vi "メイン.vi"() -> (2 "測定周期/ms":dbl, 3 "値転記用配列":T2[](array[typedef]))   [LabVIEW 2021] (continued)
                          # "csv作成の為表へクラスタ(実測値)書き込み"
                          # "⑤"
                          # "③"
                          # "④"
                          n3514 = local read "メインON/OFF_\n設定 7"() -> (w6014:T1)
                          n3515 = Unbundle By Name(w6014) -> ("使用ON/OFF"=w6010:bool)
                          n3516 = control-ref of="前回値転記用配列"() -> (w6008:refnum<vi>)
                          n3517 = local read "メイン設定_設定 7"() -> (w6015:T2)
                          n3518 = call "メイン_測定値配列_CSV転記サブ.vi"("メイン設定_設定入力"=w6015, "ループ反復数値入力"=w6012, "実測設定項目"=w6013, "使用ON/OFF"=w6010, "前回値転記用配列"=w6008) -> ("ループ反復数値出力"=w6011:i32, "メイン設定_設定出力"=w6009:T2)  [unwired: 5 in]
                          n3519 = local write "メイン設定_設定 7"(w6009) -> ()
                          n3520 = Add(x=8, y=w6011) -> (x+y=w6004:i32)
                          n3521 = Add(x=w6011, y=9) -> (x+y=w6002:i32)
                          n3522 = local read "csv作成表"() -> (w5998:string[][])
                          n3523 = Unbundle By Name(w6009) -> ("実測値(MAX)"=w6005:string, "実測値(MIN)"=w6006:string)
                          n3524 = Replace Array Subset(array=w5998, new element #1=w6005, index (row) #1=w6003, index (col) #1=w6004, new element #2=w6006, index (row) #2=w6003, index (col) #2=w6002) -> (w6000:string[][])
                          n3525 = Select(t=w6000, s=w6010, f=w5998) -> (s? t:f=w6001:string[][])
                          n3526 = local write "csv作成表"(w6001) -> ()
                        }
                        frame 7 {
                          w6021 = 2
                          # "B"
                          # "A"
                          # "csv作成の為表へクラスタ(実測値)書き込み"
                          # "⑤"
                          # "③"
                          # "④"
                          n3527 = local read "メインON/OFF_\n設定 8"() -> (w6032:T1)
                          n3528 = Unbundle By Name(w6032) -> ("使用ON/OFF"=w6028:bool)
                          n3529 = control-ref of="前回値転記用配列"() -> (w6026:refnum<vi>)
                          n3530 = local read "メイン設定_設定 8"() -> (w6033:T2)
                          n3531 = call "メイン_測定値配列_CSV転記サブ.vi"("メイン設定_設定入力"=w6033, "ループ反復数値入力"=w6030, "実測設定項目"=w6031, "使用ON/OFF"=w6028, "前回値転記用配列"=w6026) -> ("ループ反復数値出力"=w6029:i32, "メイン設定_設定出力"=w6027:T2)  [unwired: 5 in]
                          n3532 = local write "メイン設定_設定 8"(w6027) -> ()
                          n3533 = Add(x=9, y=w6029) -> (x+y=w6022:i32)
                          n3534 = Add(x=w6029, y=10) -> (x+y=w6020:i32)
                          n3535 = local read "csv作成表"() -> (w6016:string[][])
                          n3536 = Unbundle By Name(w6027) -> ("実測値(MAX)"=w6023:string, "実測値(MIN)"=w6024:string)
                          n3537 = Replace Array Subset(array=w6016, new element #1=w6023, index (row) #1=w6021, index (col) #1=w6022, new element #2=w6024, index (row) #2=w6021, index (col) #2=w6020) -> (w6018:string[][])
                          n3538 = Select(t=w6018, s=w6028, f=w6016) -> (s? t:f=w6019:string[][])
                          n3539 = local write "csv作成表"(w6019) -> ()
                        }
                        frame 8 {
                          w6039 = 2
                          # "B"
                          # "A"
                          # "csv作成の為表へクラスタ(実測値)書き込み"
                          # "⑤"
                          # "③"
                          # "④"
                          n3540 = local read "メインON/OFF_\n設定 9"() -> (w6050:T1)
                          n3541 = Unbundle By Name(w6050) -> ("使用ON/OFF"=w6046:bool)
                          n3542 = control-ref of="前回値転記用配列"() -> (w6044:refnum<vi>)
                          n3543 = local read "メイン設定_設定 9"() -> (w6051:T2)
                          n3544 = call "メイン_測定値配列_CSV転記サブ.vi"("メイン設定_設定入力"=w6051, "ループ反復数値入力"=w6048, "実測設定項目"=w6049, "使用ON/OFF"=w6046, "前回値転記用配列"=w6044) -> ("ループ反復数値出力"=w6047:i32, "メイン設定_設定出力"=w6045:T2)  [unwired: 5 in]
                          n3545 = local write "メイン設定_設定 9"(w6045) -> ()
                          n3546 = Add(x=10, y=w6047) -> (x+y=w6040:i32)
                          n3547 = Add(x=w6047, y=11) -> (x+y=w6038:i32)
                          n3548 = local read "csv作成表"() -> (w6034:string[][])
                          n3549 = Unbundle By Name(w6045) -> ("実測値(MAX)"=w6041:string, "実測値(MIN)"=w6042:string)
                          n3550 = Replace Array Subset(array=w6034, new element #1=w6041, index (row) #1=w6039, index (col) #1=w6040, new element #2=w6042, index (row) #2=w6039, index (col) #2=w6038) -> (w6036:string[][])
                          n3551 = Select(t=w6036, s=w6046, f=w6034) -> (s? t:f=w6037:string[][])
                          n3552 = local write "csv作成表"(w6037) -> ()
                        }
                        frame 9 {
                          w6057 = 2
                          # "B"
                          # "A"
                          # "csv作成の為表へクラスタ(実測値)書き込み"
                          # "⑤"
                          # "③"
                          # "④"
                          n3553 = local read "メインON/OFF_\n設定 10"() -> (w6068:T1)
                          n3554 = Unbundle By Name(w6068) -> ("使用ON/OFF"=w6064:bool)
                          n3555 = control-ref of="前回値転記用配列"() -> (w6062:refnum<vi>)
                          n3556 = local read "メイン設定_設定 10"() -> (w6069:T2)
                          n3557 = call "メイン_測定値配列_CSV転記サブ.vi"("メイン設定_設定入力"=w6069, "ループ反復数値入力"=w6066, "実測設定項目"=w6067, "使用ON/OFF"=w6064, "前回値転記用配列"=w6062) -> ("ループ反復数値出力"=w6065:i32, "メイン設定_設定出力"=w6063:T2)  [unwired: 5 in]
                          n3558 = local write "メイン設定_設定 10"(w6063) -> ()
                          n3559 = Add(x=11, y=w6065) -> (x+y=w6058:i32)
                          n3560 = Add(x=w6065, y=12) -> (x+y=w6056:i32)
                          n3561 = local read "csv作成表"() -> (w6052:string[][])
                          n3562 = Unbundle By Name(w6063) -> ("実測値(MAX)"=w6059:string, "実測値(MIN)"=w6060:string)
                          n3563 = Replace Array Subset(array=w6052, new element #1=w6059, index (row) #1=w6057, index (col) #1=w6058, new element #2=w6060, index (row) #2=w6057, index (col) #2=w6056) -> (w6054:string[][])
                          n3564 = Select(t=w6054, s=w6064, f=w6052) -> (s? t:f=w6055:string[][])
                          n3565 = local write "csv作成表"(w6055) -> ()
                        }
                        frame 10 {
                          w6075 = 2
                          # "B"
                          # "A"
                          # "csv作成の為表へクラスタ(実測値)書き込み"
                          # "⑤"
                          # "③"
                          # "④"
                          n3566 = local read "メインON/OFF_\n設定 11"() -> (w6086:T1)
                          n3567 = Unbundle By Name(w6086) -> ("使用ON/OFF"=w6082:bool)
                          n3568 = control-ref of="前回値転記用配列"() -> (w6080:refnum<vi>)
                          n3569 = local read "メイン設定_設定 11"() -> (w6087:T2)
                          n3570 = call "メイン_測定値配列_CSV転記サブ.vi"("メイン設定_設定入力"=w6087, "ループ反復数値入力"=w6084, "実測設定項目"=w6085, "使用ON/OFF"=w6082, "前回値転記用配列"=w6080) -> ("ループ反復数値出力"=w6083:i32, "メイン設定_設定出力"=w6081:T2)  [unwired: 5 in]
                          n3571 = local write "メイン設定_設定 11"(w6081) -> ()
                          n3572 = Add(x=12, y=w6083) -> (x+y=w6076:i32)
                          n3573 = Add(x=w6083, y=13) -> (x+y=w6074:i32)
                          n3574 = local read "csv作成表"() -> (w6070:string[][])
                          n3575 = Unbundle By Name(w6081) -> ("実測値(MAX)"=w6077:string, "実測値(MIN)"=w6078:string)
                          n3576 = Replace Array Subset(array=w6070, new element #1=w6077, index (row) #1=w6075, index (col) #1=w6076, new element #2=w6078, index (row) #2=w6075, index (col) #2=w6074) -> (w6072:string[][])
                          n3577 = Select(t=w6072, s=w6082, f=w6070) -> (s? t:f=w6073:string[][])
                          n3578 = local write "csv作成表"(w6073) -> ()
                        }
                        frame 11 {
                          w6093 = 2
                          # "B"
                          # "A"
                          # "csv作成の為表へクラスタ(実測値)書き込み"
                          # "⑤"
                          # "③"
                          # "④"
                          n3579 = local read "メインON/OFF_\n設定 12"() -> (w6104:T1)
                          n3580 = Unbundle By Name(w6104) -> ("使用ON/OFF"=w6100:bool)
                          n3581 = control-ref of="前回値転記用配列"() -> (w6098:refnum<vi>)
                          n3582 = local read "メイン設定_設定 12"() -> (w6105:T2)
                          n3583 = call "メイン_測定値配列_CSV転記サブ.vi"("メイン設定_設定入力"=w6105, "ループ反復数値入力"=w6102, "実測設定項目"=w6103, "使用ON/OFF"=w6100, "前回値転記用配列"=w6098) -> ("ループ反復数値出力"=w6101:i32, "メイン設定_設定出力"=w6099:T2)  [unwired: 5 in]
                          n3584 = local write "メイン設定_設定 12"(w6099) -> ()
                          n3585 = Add(x=13, y=w6101) -> (x+y=w6094:i32)
                          n3586 = Add(x=w6101, y=14) -> (x+y=w6092:i32)
                          n3587 = local read "csv作成表"() -> (w6088:string[][])
                          n3588 = Unbundle By Name(w6099) -> ("実測値(MAX)"=w6095:string, "実測値(MIN)"=w6096:string)
                          n3589 = Replace Array Subset(array=w6088, new element #1=w6095, index (row) #1=w6093, index (col) #1=w6094, new element #2=w6096, index (row) #2=w6093, index (col) #2=w6092) -> (w6090:string[][])
                          n3590 = Select(t=w6090, s=w6100, f=w6088) -> (s? t:f=w6091:string[][])
                          n3591 = local write "csv作成表"(w6091) -> ()
                        }
                      }
                    }
                  }
                }
                n3592 = local write "値転記用配列"(w5862) -> ()
                n3593 = flat-sequence {
                  tunnel: [w5877] -> w5863
                  tunnel: w5862 -> [w5877]
                  frame #0 {
                    w5872 = T9 {"Horizontal"=-51, "Vertical"=648} ("座標 9")
                    n3594 = control-ref of="このVI"() -> (w5873:refnum<vi>)
                    n3595 = property on="ペーン 2" class="Pane"("Origin"=w5872) -> ()  [unwired: 2 in, 2 out]
                    n3596 = property on="ペーン 2" class="Pane"("Origin"=w5872) -> ()  [unwired: 2 in, 2 out]
                    n3597 = control-ref of="このVI"() -> (w5875:refnum<vi>)
                    n3598 = Unbundle(w5872) -> ("Vertical"=w5874:i16)  [unwired: 1 out]
                    n3599 = Unbundle(w5872) -> ("Vertical"=w5876:i16)  [unwired: 1 out]
                    n3600 = call "メイン_装飾移動サブ.vi"("Y軸座標入力"=w5874, "VI入力"=w5873) -> ()  [unwired: 10 in]
                    n3601 = call "メイン_装飾枠移動サブ.vi"("Y軸座標入力"=w5876, "VI入力"=w5875) -> ()  [unwired: 10 in]
                  }
                }
              }
              frame #1 {
                w6107 = T8."Enabled" ("無効")
                # "⑪ボタンの無効解除"
                n3602 = for {
                  N: 12 -> [_]
                  tunnel: w6107 -> [w6110]
                  i -> [w6111]
                  n3603 = case shown="11" w6111 {
                    tunnel: w6110 -> [w6112 w6113 w6114 w6115 w6116 w6117 w6118 w6119 w6120 w6121 w6122 w6123]
                    frame 0, Default {
                      n3604 = property on="メイン測定ボタン_単発 1" class="Bool (指定)"("DisabledEnum"=w6112) -> ()  [unwired: 2 in, 2 out]
                      n3605 = property on="メイン測定ボタン_連続 1" class="Bool (指定)"("DisabledEnum"=w6112) -> ()  [unwired: 2 in, 2 out]
                    }
                    frame 1 {
                      n3606 = property on="メイン測定ボタン_単発 2" class="Bool (指定)"("DisabledEnum"=w6113) -> ()  [unwired: 2 in, 2 out]
                      n3607 = property on="メイン測定ボタン_連続 2" class="Bool (指定)"("DisabledEnum"=w6113) -> ()  [unwired: 2 in, 2 out]
                    }
                    frame 2 {
                      n3608 = property on="メイン測定ボタン_単発 3" class="Bool (指定)"("DisabledEnum"=w6114) -> ()  [unwired: 2 in, 2 out]
                      n3609 = property on="メイン測定ボタン_連続 3" class="Bool (指定)"("DisabledEnum"=w6114) -> ()  [unwired: 2 in, 2 out]
                    }
                    frame 3 {
                      n3610 = property on="メイン測定ボタン_単発 4" class="Bool (指定)"("DisabledEnum"=w6115) -> ()  [unwired: 2 in, 2 out]
                      n3611 = property on="メイン測定ボタン_連続 4" class="Bool (指定)"("DisabledEnum"=w6115) -> ()  [unwired: 2 in, 2 out]
                    }
                    frame 4 {
                      n3612 = property on="メイン測定ボタン_単発 5" class="Bool (指定)"("DisabledEnum"=w6116) -> ()  [unwired: 2 in, 2 out]
                      n3613 = property on="メイン測定ボタン_連続 5" class="Bool (指定)"("DisabledEnum"=w6116) -> ()  [unwired: 2 in, 2 out]
                    }
                    frame 5 {
                      n3614 = property on="メイン測定ボタン_連続 6" class="Bool (指定)"("DisabledEnum"=w6117) -> ()  [unwired: 2 in, 2 out]
                      n3615 = property on="メイン測定ボタン_単発 6" class="Bool (指定)"("DisabledEnum"=w6117) -> ()  [unwired: 2 in, 2 out]
                    }
                    frame 6 {
                      n3616 = property on="メイン測定ボタン_連続 7" class="Bool (指定)"("DisabledEnum"=w6118) -> ()  [unwired: 2 in, 2 out]
                      n3617 = property on="メイン測定ボタン_単発 7" class="Bool (指定)"("DisabledEnum"=w6118) -> ()  [unwired: 2 in, 2 out]
                    }
                    frame 7 {
                      n3618 = property on="メイン測定ボタン_単発 8" class="Bool (指定)"("DisabledEnum"=w6119) -> ()  [unwired: 2 in, 2 out]
                      n3619 = property on="メイン測定ボタン_連続 8" class="Bool (指定)"("DisabledEnum"=w6119) -> ()  [unwired: 2 in, 2 out]
                    }
                    frame 8 {
                      n3620 = property on="メイン測定ボタン_単発 9" class="Bool (指定)"("DisabledEnum"=w6120) -> ()  [unwired: 2 in, 2 out]
                      n3621 = property on="メイン測定ボタン_連続 9" class="Bool (指定)"("DisabledEnum"=w6120) -> ()  [unwired: 2 in, 2 out]
                    }
                    frame 9 {
                      n3622 = property on="メイン測定ボタン_単発 10" class="Bool (指定)"("DisabledEnum"=w6121) -> ()  [unwired: 2 in, 2 out]
                      n3623 = property on="メイン測定ボタン_連続 10" class="Bool (指定)"("DisabledEnum"=w6121) -> ()  [unwired: 2 in, 2 out]
                    }
                    frame 10 {
                      n3624 = property on="メイン測定ボタン_単発 11" class="Bool (指定)"("DisabledEnum"=w6122) -> ()  [unwired: 2 in, 2 out]
                      n3625 = property on="メイン測定ボタン_連続 11" class="Bool (指定)"("DisabledEnum"=w6122) -> ()  [unwired: 2 in, 2 out]
                    }
                    frame 11 {
                      n3626 = property on="メイン測定ボタン_連続 12" class="Bool (指定)"("DisabledEnum"=w6123) -> ()  [unwired: 2 in, 2 out]
                      n3627 = property on="メイン測定ボタン_単発 12" class="Bool (指定)"("DisabledEnum"=w6123) -> ()  [unwired: 2 in, 2 out]
                    }
                  }
                }
                n3628 = local write "測定新値\nリセット用 10"(TRUE) -> ()
                n3629 = property on="TOPページへ" class="Bool"("DisabledEnum"=w6107) -> ()  [unwired: 2 in, 2 out]
                n3630 = property on="保存して終了" class="Bool"("DisabledEnum"=w6107) -> ()  [unwired: 2 in, 2 out]
                n3631 = property on="保存せずに" class="Bool"("DisabledEnum"=w6107) -> ()  [unwired: 2 in, 2 out]
              }
            }
          }
          frame True {
          }
        }
      }
      frame "測定11" {
        # "⑦"
        # "項目別のボタンで測定を行う為、項目分必要"
        n3632 = local read "測定旧値 11"() -> (w6127:bool)
        n3633 = case shown="FALSE" w6127 {
          tunnel: w6125 -> [w6130 w6393]
          tunnel: [w6129 w6393] -> w6126
          frame False {
            n3634 = flat-sequence {
              tunnel: w6130 -> [w6140]
              tunnel: [w6132] -> w6128
              tunnel: [w6378] -> w6129
              tunnel: w6128 -> [w6378]
              frame #0 {
                # "※複製コピー時変更する項目\n①②\nローカル変数\n\n入れ子のケースストラクチャ\"2\"を複製\n\n0～数だけ変更する\n③④⑤\nローカル変数\n\n※AB\n行番号の変更をする必要がある\n\n--------------------------------\nこの後イベントストラクチャ複製する\n--------------------------------\nイベントストラクチャ複製後\n\n⑦⑧\nローカル変数\n⑨\n装飾体の位置設定\n-51は固定\n前ケースの数値+72\n⑩\n測定新値リセット用\nのボタンが複製されているので、\nフロントパネルを整理する\n⑪\nプロパティノード\nボタンの無効解除クリア以外全てのボタン対象"
                # "実測完了の簡易疑似コード\n\n1)測定モードが単発・連続、多点かで転記する配列を変える\n2)値転記用配列へ転記\n\nここからゲージ分を繰り返す必要がある\n\n3)配列0を取り出す\n4)配列0のポートNoを取り出す\n5)メイン測定_設定配列(測定1の対象配列)のポートNoと比較\n6)同じだったら処理をする。違ったら何もしない\n7)同じだったら配列0のメインON/OFF_設定1の使用ON/OFFがTrueかFalseか\nFlaseだったら前回値転記用配列から前回の値をメイン設定_設定へ転記\nTrueだったらメイン設定_設定の測定モードから\n0単発、1連続、3多点\nの処理を行う\n8)測定値をメイン設定_設定へ転記したら、前回転記用配列へ転記する"
                # "⑨"
                # "⑧"
                # "②"
                # "グループNO(表示上はポートNo)が同じだったら値を転記する\n\n測定した配列のグループNOと値転記用配列の他の指標グループNOを比較する\n＝だったら、対象の配列のON/OFFボタンがTrueか確認し、\nTrueだったら、測定モードによって、値かMAX、MINの数値を転記する\n\nグループNOが同じでなければ、転記しない(何もしない)"
                # "まず値転記用配列に測定の値を転記"
                # "実測定画面vi動作"
                n3635 = local read "メイン設定_設定 11"() -> (w6135:T2)
                n3636 = local read "測定新値 11"() -> (→"測定新値\nリセット用 11":bool)
                n3637 = local read "測定周期/ms"() -> (w6133:dbl)
                n3638 = Unbundle By Name(w6135) -> ("測定モード"=w6136:u16)
                n3639 = call "実測定画面.vi"("実測設定項目配列_\nメインからの転記"=w6140, "測定周期/ms_制御器"=w6133) -> ("実測設定項目配列_\nゲージIOへ転記用"=w6138:T2[], "実測設定項目配列_\n多点測定メイン転記用"=w6137:T2[])  [unwired: 11 in, 1 out]
                n3640 = case shown="1" w6136 {
                  tunnel: w6138 -> [w6147 w6148 _]
                  tunnel: [w6147 w6148 w6149] -> w6131
                  tunnel: w6137 -> [_ _ w6149]
                  frame 0, Default {
                  }
                  frame 1 {
                  }
                  frame 2 {
                  }
                }
                n3641 = for {
                  N: 32 -> [_]
                  tunnel: w6131 -> [w6156]
                  i -> [w6151]
                  # "①"
                  # "※複製コピーはこのケースで行う"
                  # "32回分"
                  # "比較する固定GNO"
                  n3642 = local read "メイン設定_設定 11"() -> (w6150:T2)
                  n3643 = Index Array(array=w6156, index=w6151) -> (element=w6155:T2)
                  n3644 = Unbundle By Name(w6150) -> ("ポートNo."=w6154:dbl)
                  n3645 = Unbundle By Name(w6155) -> ("ポートNo."=w6153:dbl)
                  n3646 = Equal?(x=w6154, y=w6153) -> (x = y?=w6152:bool)
                  n3647 = case shown="TRUE" w6152 {
                    tunnel: w6155 -> [_ w6158]
                    tunnel: w6151 -> [_ w6157]
                    frame False {
                    }
                    frame True {
                      n3648 = case shown="0, デフォルト" w6157 {
                        tunnel: w6158 -> [w6174 w6192 w6210 w6228 w6246 w6264 w6282 w6300 w6318 w6336 w6354 w6372]
                        tunnel: w6157 -> [w6173 w6191 w6209 w6227 w6245 w6263 w6281 w6299 w6317 w6335 w6353 w6371]
                        frame 0, Default {
                          w6164 = 2
                          # "B"
                          # "A"
                          # "csv作成の為表へクラスタ(実測値)書き込み"
                          # "⑤"
                          # "③"
                          # "④"
                          n3649 = local read "メインON/OFF_\n設定 1"() -> (w6175:T1)
                          n3650 = Unbundle By Name(w6175) -> ("使用ON/OFF"=w6171:bool)
                          n3651 = control-ref of="前回値転記用配列"() -> (w6169:refnum<vi>)
                          n3652 = local read "メイン設定_設定 1"() -> (w6176:T2)
                          n3653 = call "メイン_測定値配列_CSV転記サブ.vi"("メイン設定_設定入力"=w6176, "ループ反復数値入力"=w6173, "実測設定項目"=w6174, "使用ON/OFF"=w6171, "前回値転記用配列"=w6169) -> ("ループ反復数値出力"=w6172:i32, "メイン設定_設定出力"=w6170:T2)  [unwired: 5 in]
                          n3654 = local write "メイン設定_設定 1"(w6170) -> ()
                          n3655 = Add(x=2, y=w6172) -> (x+y=w6165:i32)
                          n3656 = Add(x=w6172, y=3) -> (x+y=w6163:i32)
                          n3657 = local read "csv作成表"() -> (w6159:string[][])
                          n3658 = Unbundle By Name(w6170) -> ("実測値(MAX)"=w6166:string, "実測値(MIN)"=w6167:string)
                          n3659 = Replace Array Subset(array=w6159, new element #1=w6166, index (row) #1=w6164, index (col) #1=w6165, new element #2=w6167, index (row) #2=w6164, index (col) #2=w6163) -> (w6161:string[][])
                          n3660 = Select(t=w6161, s=w6171, f=w6159) -> (s? t:f=w6162:string[][])
                          n3661 = local write "csv作成表"(w6162) -> ()
                        }
                        frame 1 {
                          w6182 = 2
                          # "B"
                          # "A"
                          # "csv作成の為表へクラスタ(実測値)書き込み"
                          # "⑤"
                          # "③"
                          # "④"
                          n3662 = local read "メインON/OFF_\n設定 2"() -> (w6193:T1)
                          n3663 = Unbundle By Name(w6193) -> ("使用ON/OFF"=w6189:bool)
                          n3664 = control-ref of="前回値転記用配列"() -> (w6187:refnum<vi>)
                          n3665 = local read "メイン設定_設定 2"() -> (w6194:T2)
                          n3666 = call "メイン_測定値配列_CSV転記サブ.vi"("メイン設定_設定入力"=w6194, "ループ反復数値入力"=w6191, "実測設定項目"=w6192, "使用ON/OFF"=w6189, "前回値転記用配列"=w6187) -> ("ループ反復数値出力"=w6190:i32, "メイン設定_設定出力"=w6188:T2)  [unwired: 5 in]
                          n3667 = local write "メイン設定_設定 2"(w6188) -> ()
                          n3668 = Add(x=3, y=w6190) -> (x+y=w6183:i32)
                          n3669 = Add(x=w6190, y=4) -> (x+y=w6181:i32)
                          n3670 = local read "csv作成表"() -> (w6177:string[][])
                          n3671 = Unbundle By Name(w6188) -> ("実測値(MAX)"=w6184:string, "実測値(MIN)"=w6185:string)
                          n3672 = Replace Array Subset(array=w6177, new element #1=w6184, index (row) #1=w6182, index (col) #1=w6183, new element #2=w6185, index (row) #2=w6182, index (col) #2=w6181) -> (w6179:string[][])
                          n3673 = Select(t=w6179, s=w6189, f=w6177) -> (s? t:f=w6180:string[][])
                          n3674 = local write "csv作成表"(w6180) -> ()
                        }
                        frame 2 {
                          w6200 = 2
                          # "B"
                          # "A"
                          # "csv作成の為表へクラスタ(実測値)書き込み"
                          # "⑤"
                          # "③"
                          # "④"
                          n3675 = local read "メインON/OFF_\n設定 3"() -> (w6211:T1)
                          n3676 = Unbundle By Name(w6211) -> ("使用ON/OFF"=w6207:bool)
                          n3677 = control-ref of="前回値転記用配列"() -> (w6205:refnum<vi>)
                          n3678 = local read "メイン設定_設定 3"() -> (w6212:T2)
                          n3679 = call "メイン_測定値配列_CSV転記サブ.vi"("メイン設定_設定入力"=w6212, "ループ反復数値入力"=w6209, "実測設定項目"=w6210, "使用ON/OFF"=w6207, "前回値転記用配列"=w6205) -> ("ループ反復数値出力"=w6208:i32, "メイン設定_設定出力"=w6206:T2)  [unwired: 5 in]
                          n3680 = local write "メイン設定_設定 3"(w6206) -> ()
                          n3681 = Add(x=4, y=w6208) -> (x+y=w6201:i32)
                          n3682 = Add(x=w6208, y=5) -> (x+y=w6199:i32)
                          n3683 = local read "csv作成表"() -> (w6195:string[][])
                          n3684 = Unbundle By Name(w6206) -> ("実測値(MAX)"=w6202:string, "実測値(MIN)"=w6203:string)
                          n3685 = Replace Array Subset(array=w6195, new element #1=w6202, index (row) #1=w6200, index (col) #1=w6201, new element #2=w6203, index (row) #2=w6200, index (col) #2=w6199) -> (w6197:string[][])
                          n3686 = Select(t=w6197, s=w6207, f=w6195) -> (s? t:f=w6198:string[][])
                          n3687 = local write "csv作成表"(w6198) -> ()
                        }
                        frame 3 {
                          w6218 = 2
                          # "B"
                          # "A"
                          # "csv作成の為表へクラスタ(実測値)書き込み"
                          # "⑤"
                          # "③"
                          # "④"
                          n3688 = local read "メインON/OFF_\n設定 4"() -> (w6229:T1)
                          n3689 = Unbundle By Name(w6229) -> ("使用ON/OFF"=w6225:bool)
                          n3690 = control-ref of="前回値転記用配列"() -> (w6223:refnum<vi>)
                          n3691 = local read "メイン設定_設定 4"() -> (w6230:T2)
                          n3692 = call "メイン_測定値配列_CSV転記サブ.vi"("メイン設定_設定入力"=w6230, "ループ反復数値入力"=w6227, "実測設定項目"=w6228, "使用ON/OFF"=w6225, "前回値転記用配列"=w6223) -> ("ループ反復数値出力"=w6226:i32, "メイン設定_設定出力"=w6224:T2)  [unwired: 5 in]
                          n3693 = local write "メイン設定_設定 4"(w6224) -> ()
                          n3694 = Add(x=5, y=w6226) -> (x+y=w6219:i32)
                          n3695 = Add(x=w6226, y=6) -> (x+y=w6217:i32)
                          n3696 = local read "csv作成表"() -> (w6213:string[][])
                          n3697 = Unbundle By Name(w6224) -> ("実測値(MAX)"=w6220:string, "実測値(MIN)"=w6221:string)
                          n3698 = Replace Array Subset(array=w6213, new element #1=w6220, index (row) #1=w6218, index (col) #1=w6219, new element #2=w6221, index (row) #2=w6218, index (col) #2=w6217) -> (w6215:string[][])
                          n3699 = Select(t=w6215, s=w6225, f=w6213) -> (s? t:f=w6216:string[][])
                          n3700 = local write "csv作成表"(w6216) -> ()
                        }
                        frame 4 {
                          w6236 = 2
                          # "B"
                          # "A"
                          # "csv作成の為表へクラスタ(実測値)書き込み"
                          # "⑤"
                          # "③"
                          # "④"
                          n3701 = local read "メインON/OFF_\n設定 5"() -> (w6247:T1)
                          n3702 = Unbundle By Name(w6247) -> ("使用ON/OFF"=w6243:bool)
                          n3703 = control-ref of="前回値転記用配列"() -> (w6241:refnum<vi>)
                          n3704 = local read "メイン設定_設定 5"() -> (w6248:T2)
                          n3705 = call "メイン_測定値配列_CSV転記サブ.vi"("メイン設定_設定入力"=w6248, "ループ反復数値入力"=w6245, "実測設定項目"=w6246, "使用ON/OFF"=w6243, "前回値転記用配列"=w6241) -> ("ループ反復数値出力"=w6244:i32, "メイン設定_設定出力"=w6242:T2)  [unwired: 5 in]
                          n3706 = local write "メイン設定_設定 5"(w6242) -> ()
                          n3707 = Add(x=6, y=w6244) -> (x+y=w6237:i32)
                          n3708 = Add(x=w6244, y=7) -> (x+y=w6235:i32)
                          n3709 = local read "csv作成表"() -> (w6231:string[][])
                          n3710 = Unbundle By Name(w6242) -> ("実測値(MAX)"=w6238:string, "実測値(MIN)"=w6239:string)
                          n3711 = Replace Array Subset(array=w6231, new element #1=w6238, index (row) #1=w6236, index (col) #1=w6237, new element #2=w6239, index (row) #2=w6236, index (col) #2=w6235) -> (w6233:string[][])
                          n3712 = Select(t=w6233, s=w6243, f=w6231) -> (s? t:f=w6234:string[][])
                          n3713 = local write "csv作成表"(w6234) -> ()
                        }
                        frame 5 {
                          w6254 = 2
                          # "B"
                          # "A"
                          # "csv作成の為表へクラスタ(実測値)書き込み"
                          # "⑤"
                          # "③"
                          # "④"
                          n3714 = local read "メインON/OFF_\n設定 6"() -> (w6265:T1)
                          n3715 = Unbundle By Name(w6265) -> ("使用ON/OFF"=w6261:bool)
                          n3716 = control-ref of="前回値転記用配列"() -> (w6259:refnum<vi>)
                          n3717 = local read "メイン設定_設定 6"() -> (w6266:T2)
                          n3718 = call "メイン_測定値配列_CSV転記サブ.vi"("メイン設定_設定入力"=w6266, "ループ反復数値入力"=w6263, "実測設定項目"=w6264, "使用ON/OFF"=w6261, "前回値転記用配列"=w6259) -> ("ループ反復数値出力"=w6262:i32, "メイン設定_設定出力"=w6260:T2)  [unwired: 5 in]
                          n3719 = local write "メイン設定_設定 6"(w6260) -> ()
                          n3720 = Add(x=7, y=w6262) -> (x+y=w6255:i32)
                          n3721 = Add(x=w6262, y=8) -> (x+y=w6253:i32)
                          n3722 = local read "csv作成表"() -> (w6249:string[][])
                          n3723 = Unbundle By Name(w6260) -> ("実測値(MAX)"=w6256:string, "実測値(MIN)"=w6257:string)
                          n3724 = Replace Array Subset(array=w6249, new element #1=w6256, index (row) #1=w6254, index (col) #1=w6255, new element #2=w6257, index (row) #2=w6254, index (col) #2=w6253) -> (w6251:string[][])
                          n3725 = Select(t=w6251, s=w6261, f=w6249) -> (s? t:f=w6252:string[][])
                          n3726 = local write "csv作成表"(w6252) -> ()
                        }
                        frame 6 {
                          w6272 = 2
                          # "B"
                          # "A"
                          # "csv作成の為表へクラスタ(実測値)書き込み"
                          # "⑤"
                          # "③"
                          # "④"
                          n3727 = local read "メインON/OFF_\n設定 7"() -> (w6283:T1)
                          n3728 = Unbundle By Name(w6283) -> ("使用ON/OFF"=w6279:bool)
                          n3729 = control-ref of="前回値転記用配列"() -> (w6277:refnum<vi>)
                          n3730 = local read "メイン設定_設定 7"() -> (w6284:T2)
                          n3731 = call "メイン_測定値配列_CSV転記サブ.vi"("メイン設定_設定入力"=w6284, "ループ反復数値入力"=w6281, "実測設定項目"=w6282, "使用ON/OFF"=w6279, "前回値転記用配列"=w6277) -> ("ループ反復数値出力"=w6280:i32, "メイン設定_設定出力"=w6278:T2)  [unwired: 5 in]
                          n3732 = local write "メイン設定_設定 7"(w6278) -> ()
                          n3733 = Add(x=8, y=w6280) -> (x+y=w6273:i32)
                          n3734 = Add(x=w6280, y=9) -> (x+y=w6271:i32)
                          n3735 = local read "csv作成表"() -> (w6267:string[][])
                          n3736 = Unbundle By Name(w6278) -> ("実測値(MAX)"=w6274:string, "実測値(MIN)"=w6275:string)
                          n3737 = Replace Array Subset(array=w6267, new element #1=w6274, index (row) #1=w6272, index (col) #1=w6273, new element #2=w6275, index (row) #2=w6272, index (col) #2=w6271) -> (w6269:string[][])
                          n3738 = Select(t=w6269, s=w6279, f=w6267) -> (s? t:f=w6270:string[][])
                          n3739 = local write "csv作成表"(w6270) -> ()
                        }
                        frame 7 {
                          w6290 = 2
                          # "B"
                          # "A"
                          # "csv作成の為表へクラスタ(実測値)書き込み"
                          # "⑤"
                          # "③"
                          # "④"
                          n3740 = local read "メインON/OFF_\n設定 8"() -> (w6301:T1)
                          n3741 = Unbundle By Name(w6301) -> ("使用ON/OFF"=w6297:bool)
                          n3742 = control-ref of="前回値転記用配列"() -> (w6295:refnum<vi>)
                          n3743 = local read "メイン設定_設定 8"() -> (w6302:T2)
                          n3744 = call "メイン_測定値配列_CSV転記サブ.vi"("メイン設定_設定入力"=w6302, "ループ反復数値入力"=w6299, "実測設定項目"=w6300, "使用ON/OFF"=w6297, "前回値転記用配列"=w6295) -> ("ループ反復数値出力"=w6298:i32, "メイン設定_設定出力"=w6296:T2)  [unwired: 5 in]
                          n3745 = local write "メイン設定_設定 8"(w6296) -> ()
                          n3746 = Add(x=9, y=w6298) -> (x+y=w6291:i32)
                          n3747 = Add(x=w6298, y=10) -> (x+y=w6289:i32)
                          n3748 = local read "csv作成表"() -> (w6285:string[][])
                          n3749 = Unbundle By Name(w6296) -> ("実測値(MAX)"=w6292:string, "実測値(MIN)"=w6293:string)
                          n3750 = Replace Array Subset(array=w6285, new element #1=w6292, index (row) #1=w6290, index (col) #1=w6291, new element #2=w6293, index (row) #2=w6290, index (col) #2=w6289) -> (w6287:string[][])
                          n3751 = Select(t=w6287, s=w6297, f=w6285) -> (s? t:f=w6288:string[][])
                          n3752 = local write "csv作成表"(w6288) -> ()
                        }
                        frame 8 {
                          w6308 = 2
                          # "B"
                          # "A"
                          # "csv作成の為表へクラスタ(実測値)書き込み"
                          # "⑤"
                          # "③"
                          # "④"
                          n3753 = local read "メインON/OFF_\n設定 9"() -> (w6319:T1)
                          n3754 = Unbundle By Name(w6319) -> ("使用ON/OFF"=w6315:bool)
                          n3755 = control-ref of="前回値転記用配列"() -> (w6313:refnum<vi>)
                          n3756 = local read "メイン設定_設定 9"() -> (w6320:T2)
                          n3757 = call "メイン_測定値配列_CSV転記サブ.vi"("メイン設定_設定入力"=w6320, "ループ反復数値入力"=w6317, "実測設定項目"=w6318, "使用ON/OFF"=w6315, "前回値転記用配列"=w6313) -> ("ループ反復数値出力"=w6316:i32, "メイン設定_設定出力"=w6314:T2)  [unwired: 5 in]
                          n3758 = local write "メイン設定_設定 9"(w6314) -> ()
                          n3759 = Add(x=10, y=w6316) -> (x+y=w6309:i32)
                          n3760 = Add(x=w6316, y=11) -> (x+y=w6307:i32)
                          n3761 = local read "csv作成表"() -> (w6303:string[][])
                          n3762 = Unbundle By Name(w6314) -> ("実測値(MAX)"=w6310:string, "実測値(MIN)"=w6311:string)
                          n3763 = Replace Array Subset(array=w6303, new element #1=w6310, index (row) #1=w6308, index (col) #1=w6309, new element #2=w6311, index (row) #2=w6308, index (col) #2=w6307) -> (w6305:string[][])
                          n3764 = Select(t=w6305, s=w6315, f=w6303) -> (s? t:f=w6306:string[][])
                          n3765 = local write "csv作成表"(w6306) -> ()
                        }
                        frame 9 {
                          w6326 = 2
                          # "B"
                          # "A"
                          # "csv作成の為表へクラスタ(実測値)書き込み"
                          # "⑤"
                          # "③"
                          # "④"
                          n3766 = local read "メインON/OFF_\n設定 10"() -> (w6337:T1)
                          n3767 = Unbundle By Name(w6337) -> ("使用ON/OFF"=w6333:bool)
                          n3768 = control-ref of="前回値転記用配列"() -> (w6331:refnum<vi>)
                          n3769 = local read "メイン設定_設定 10"() -> (w6338:T2)
                          n3770 = call "メイン_測定値配列_CSV転記サブ.vi"("メイン設定_設定入力"=w6338, "ループ反復数値入力"=w6335, "実測設定項目"=w6336, "使用ON/OFF"=w6333, "前回値転記用配列"=w6331) -> ("ループ反復数値出力"=w6334:i32, "メイン設定_設定出力"=w6332:T2)  [unwired: 5 in]
                          n3771 = local write "メイン設定_設定 10"(w6332) -> ()
                          n3772 = Add(x=11, y=w6334) -> (x+y=w6327:i32)
                          n3773 = Add(x=w6334, y=12) -> (x+y=w6325:i32)
                          n3774 = local read "csv作成表"() -> (w6321:string[][])
                          n3775 = Unbundle By Name(w6332) -> ("実測値(MAX)"=w6328:string, "実測値(MIN)"=w6329:string)
                          n3776 = Replace Array Subset(array=w6321, new element #1=w6328, index (row) #1=w6326, index (col) #1=w6327, new element #2=w6329, index (row) #2=w6326, index (col) #2=w6325) -> (w6323:string[][])
                          n3777 = Select(t=w6323, s=w6333, f=w6321) -> (s? t:f=w6324:string[][])
                          n3778 = local write "csv作成表"(w6324) -> ()
                        }
                        frame 10 {
                          w6344 = 2
                          # "B"
                          # "A"
                          # "csv作成の為表へクラスタ(実測値)書き込み"
                          # "⑤"
                          # "③"
                          # "④"
                          n3779 = local read "メインON/OFF_\n設定 11"() -> (w6355:T1)
                          n3780 = Unbundle By Name(w6355) -> ("使用ON/OFF"=w6351:bool)
                          n3781 = control-ref of="前回値転記用配列"() -> (w6349:refnum<vi>)
                          n3782 = local read "メイン設定_設定 11"() -> (w6356:T2)
                          n3783 = call "メイン_測定値配列_CSV転記サブ.vi"("メイン設定_設定入力"=w6356, "ループ反復数値入力"=w6353, "実測設定項目"=w6354, "使用ON/OFF"=w6351, "前回値転記用配列"=w6349) -> ("ループ反復数値出力"=w6352:i32, "メイン設定_設定出力"=w6350:T2)  [unwired: 5 in]
                          n3784 = local write "メイン設定_設定 11"(w6350) -> ()
                          n3785 = Add(x=12, y=w6352) -> (x+y=w6345:i32)
                          n3786 = Add(x=w6352, y=13) -> (x+y=w6343:i32)
                          n3787 = local read "csv作成表"() -> (w6339:string[][])
                          n3788 = Unbundle By Name(w6350) -> ("実測値(MAX)"=w6346:string, "実測値(MIN)"=w6347:string)
                          n3789 = Replace Array Subset(array=w6339, new element #1=w6346, index (row) #1=w6344, index (col) #1=w6345, new element #2=w6347, index (row) #2=w6344, index (col) #2=w6343) -> (w6341:string[][])
                          n3790 = Select(t=w6341, s=w6351, f=w6339) -> (s? t:f=w6342:string[][])
                          n3791 = local write "csv作成表"(w6342) -> ()
                        }
                        frame 11 {
                          w6362 = 2
                          # "B"
                          # "A"
                          # "csv作成の為表へクラスタ(実測値)書き込み"
                          # "⑤"
                          # "③"
                          # "④"
                          n3792 = local read "メインON/OFF_\n設定 12"() -> (w6373:T1)
                          n3793 = Unbundle By Name(w6373) -> ("使用ON/OFF"=w6369:bool)
                          n3794 = control-ref of="前回値転記用配列"() -> (w6367:refnum<vi>)
                          n3795 = local read "メイン設定_設定 12"() -> (w6374:T2)
                          n3796 = call "メイン_測定値配列_CSV転記サブ.vi"("メイン設定_設定入力"=w6374, "ループ反復数値入力"=w6371, "実測設定項目"=w6372, "使用ON/OFF"=w6369, "前回値転記用配列"=w6367) -> ("ループ反復数値出力"=w6370:i32, "メイン設定_設定出力"=w6368:T2)  [unwired: 5 in]
                          n3797 = local write "メイン設定_設定 12"(w6368) -> ()
                          n3798 = Add(x=13, y=w6370) -> (x+y=w6363:i32)
                          n3799 = Add(x=w6370, y=14) -> (x+y=w6361:i32)
                          n3800 = local read "csv作成表"() -> (w6357:string[][])
                          n3801 = Unbundle By Name(w6368) -> ("実測値(MAX)"=w6364:string, "実測値(MIN)"=w6365:string)
                          n3802 = Replace Array Subset(array=w6357, new element #1=w6364, index (row) #1=w6362, index (col) #1=w6363, new element #2=w6365, index (row) #2=w6362, index (col) #2=w6361) -> (w6359:string[][])
                          n3803 = Select(t=w6359, s=w6369, f=w6357) -> (s? t:f=w6360:string[][])
                          n3804 = local write "csv作成表"(w6360) -> ()
                        }
                      }
                    }
                  }
                }
                n3805 = local write "値転記用配列"(w6131) -> ()
                n3806 = flat-sequence {
                  tunnel: [w6146] -> w6132
                  tunnel: w6131 -> [w6146]
                  frame #0 {
                    w6141 = T9 {"Horizontal"=-51, "Vertical"=720} ("座標 10")
                    n3807 = control-ref of="このVI"() -> (w6142:refnum<vi>)
                    n3808 = property on="ペーン 2" class="Pane"("Origin"=w6141) -> ()  [unwired: 2 in, 2 out]
                    n3809 = property on="ペーン 2" class="Pane"("Origin"=w6141) -> ()  [unwired: 2 in, 2 out]
                    n3810 = control-ref of="このVI"() -> (w6144:refnum<vi>)
                    n3811 = Unbundle(w6141) -> ("Vertical"=w6143:i16)  [unwired: 1 out]
                    n3812 = Unbundle(w6141) -> ("Vertical"=w6145:i16)  [unwired: 1 out]
                    n3813 = call "メイン_装飾移動サブ.vi"("Y軸座標入力"=w6143, "VI入力"=w6142) -> ()  [unwired: 10 in]
                    n3814 = call "メイン_装飾枠移動サブ.vi"("Y軸座標入力"=w6145, "VI入力"=w6144) -> ()  [unwired: 10 in]
                  }
                }
              }
              frame #1 {
                w6376 = T8."Enabled" ("無効")
                # "⑪ボタンの無効解除"
                n3815 = local write "測定新値\nリセット用 11"(TRUE) -> ()
                n3816 = for {
                  N: 12 -> [_]
                  tunnel: w6376 -> [w6379]
                  i -> [w6380]
                  n3817 = case shown="11" w6380 {
                    tunnel: w6379 -> [w6381 w6382 w6383 w6384 w6385 w6386 w6387 w6388 w6389 w6390 w6391 w6392]
                    frame 0, Default {
                      n3818 = property on="メイン測定ボタン_単発 1" class="Bool (指定)"("DisabledEnum"=w6381) -> ()  [unwired: 2 in, 2 out]
                      n3819 = property on="メイン測定ボタン_連続 1" class="Bool (指定)"("DisabledEnum"=w6381) -> ()  [unwired: 2 in, 2 out]
                    }
                    frame 1 {
                      n3820 = property on="メイン測定ボタン_単発 2" class="Bool (指定)"("DisabledEnum"=w6382) -> ()  [unwired: 2 in, 2 out]
                      n3821 = property on="メイン測定ボタン_連続 2" class="Bool (指定)"("DisabledEnum"=w6382) -> ()  [unwired: 2 in, 2 out]
                    }
                    frame 2 {
                      n3822 = property on="メイン測定ボタン_単発 3" class="Bool (指定)"("DisabledEnum"=w6383) -> ()  [unwired: 2 in, 2 out]
                      n3823 = property on="メイン測定ボタン_連続 3" class="Bool (指定)"("DisabledEnum"=w6383) -> ()  [unwired: 2 in, 2 out]
                    }
                    frame 3 {
                      n3824 = property on="メイン測定ボタン_単発 4" class="Bool (指定)"("DisabledEnum"=w6384) -> ()  [unwired: 2 in, 2 out]
                      n3825 = property on="メイン測定ボタン_連続 4" class="Bool (指定)"("DisabledEnum"=w6384) -> ()  [unwired: 2 in, 2 out]
                    }
                    frame 4 {
                      n3826 = property on="メイン測定ボタン_単発 5" class="Bool (指定)"("DisabledEnum"=w6385) -> ()  [unwired: 2 in, 2 out]
                      n3827 = property on="メイン測定ボタン_連続 5" class="Bool (指定)"("DisabledEnum"=w6385) -> ()  [unwired: 2 in, 2 out]
                    }
                    frame 5 {
                      n3828 = property on="メイン測定ボタン_連続 6" class="Bool (指定)"("DisabledEnum"=w6386) -> ()  [unwired: 2 in, 2 out]
                      n3829 = property on="メイン測定ボタン_単発 6" class="Bool (指定)"("DisabledEnum"=w6386) -> ()  [unwired: 2 in, 2 out]
                    }
                    frame 6 {
                      n3830 = property on="メイン測定ボタン_連続 7" class="Bool (指定)"("DisabledEnum"=w6387) -> ()  [unwired: 2 in, 2 out]
                      n3831 = property on="メイン測定ボタン_単発 7" class="Bool (指定)"("DisabledEnum"=w6387) -> ()  [unwired: 2 in, 2 out]
                    }
                    frame 7 {
                      n3832 = property on="メイン測定ボタン_単発 8" class="Bool (指定)"("DisabledEnum"=w6388) -> ()  [unwired: 2 in, 2 out]
                      n3833 = property on="メイン測定ボタン_連続 8" class="Bool (指定)"("DisabledEnum"=w6388) -> ()  [unwired: 2 in, 2 out]
                    }
                    frame 8 {
                      n3834 = property on="メイン測定ボタン_単発 9" class="Bool (指定)"("DisabledEnum"=w6389) -> ()  [unwired: 2 in, 2 out]
                      n3835 = property on="メイン測定ボタン_連続 9" class="Bool (指定)"("DisabledEnum"=w6389) -> ()  [unwired: 2 in, 2 out]
                    }
                    frame 9 {
                      n3836 = property on="メイン測定ボタン_単発 10" class="Bool (指定)"("DisabledEnum"=w6390) -> ()  [unwired: 2 in, 2 out]
                      n3837 = property on="メイン測定ボタン_連続 10" class="Bool (指定)"("DisabledEnum"=w6390) -> ()  [unwired: 2 in, 2 out]
                    }
                    frame 10 {
                      n3838 = property on="メイン測定ボタン_単発 11" class="Bool (指定)"("DisabledEnum"=w6391) -> ()  [unwired: 2 in, 2 out]
                      n3839 = property on="メイン測定ボタン_連続 11" class="Bool (指定)"("DisabledEnum"=w6391) -> ()  [unwired: 2 in, 2 out]
                    }
                    frame 11 {
                      n3840 = property on="メイン測定ボタン_連続 12" class="Bool (指定)"("DisabledEnum"=w6392) -> ()  [unwired: 2 in, 2 out]
                      n3841 = property on="メイン測定ボタン_単発 12" class="Bool (指定)"("DisabledEnum"=w6392) -> ()  [unwired: 2 in, 2 out]
                    }
                  }
                }
                n3842 = property on="TOPページへ" class="Bool"("DisabledEnum"=w6376) -> ()  [unwired: 2 in, 2 out]
                n3843 = property on="保存して終了" class="Bool"("DisabledEnum"=w6376) -> ()  [unwired: 2 in, 2 out]
                n3844 = property on="保存せずに" class="Bool"("DisabledEnum"=w6376) -> ()  [unwired: 2 in, 2 out]
              }
            }
          }
          frame True {
          }
        }
      }
      frame "測定12" {
        # "⑦"
        # "項目別のボタンで測定を行う為、項目分必要"
        n3845 = local read "測定旧値 12"() -> (w6396:bool)
        n3846 = case shown="FALSE" w6396 {
          tunnel: w6394 -> [w6399 w6662]
          tunnel: [w6398 w6662] -> w6395
          frame False {
            n3847 = flat-sequence {
              tunnel: w6399 -> [w6409]
              tunnel: [w6401] -> w6397
              tunnel: [w6647] -> w6398
              tunnel: w6397 -> [w6647]
              frame #0 {
                # "※複製コピー時変更する項目\n①②\nローカル変数\n\n入れ子のケースストラクチャ\"2\"を複製\n\n0～数だけ変更する\n③④⑤\nローカル変数\n\n※AB\n行番号の変更をする必要がある\n\n--------------------------------\nこの後イベントストラクチャ複製する\n--------------------------------\nイベントストラクチャ複製後\n\n⑦⑧\nローカル変数\n⑨\n装飾体の位置設定\n-51は固定\n前ケースの数値+72\n⑩\n測定新値リセット用\nのボタンが複製されているので、\nフロントパネルを整理する\n⑪\nプロパティノード\nボタンの無効解除クリア以外全てのボタン対象"
                # "実測完了の簡易疑似コード\n\n1)測定モードが単発・連続、多点かで転記する配列を変える\n2)値転記用配列へ転記\n\nここからゲージ分を繰り返す必要がある\n\n3)配列0を取り出す\n4)配列0のポートNoを取り出す\n5)メイン測定_設定配列(測定1の対象配列)のポートNoと比較\n6)同じだったら処理をする。違ったら何もしない\n7)同じだったら配列0のメインON/OFF_設定1の使用ON/OFFがTrueかFalseか\nFlaseだったら前回値転記用配列から前回の値をメイン設定_設定へ転記\nTrueだったらメイン設定_設定の測定モードから\n0単発、1連続、3多点\nの処理を行う\n8)測定値をメイン設定_設定へ転記したら、前回転記用配列へ転記する"
                # "⑨"
                # "⑧"
                # "②"
                # "グループNO(表示上はポートNo)が同じだったら値を転記する\n\n測定した配列のグループNOと値転記用配列の他の指標グループNOを比較する\n＝だったら、対象の配列のON/OFFボタンがTrueか確認し、\nTrueだったら、測定モードによって、値かMAX、MINの数値を転記する\n\nグループNOが同じでなければ、転記しない(何もしない)"
                # "まず値転記用配列に測定の値を転記"
                # "実測定画面vi動作"
                n3848 = local read "メイン設定_設定 12"() -> (w6404:T2)
                n3849 = local read "測定新値 12"() -> (→"測定新値\nリセット用 12":bool)
                n3850 = local read "測定周期/ms"() -> (w6402:dbl)
                n3851 = Unbundle By Name(w6404) -> ("測定モード"=w6405:u16)
                n3852 = call "実測定画面.vi"("実測設定項目配列_\nメインからの転記"=w6409, "測定周期/ms_制御器"=w6402) -> ("実測設定項目配列_\nゲージIOへ転記用"=w6407:T2[], "実測設定項目配列_\n多点測定メイン転記用"=w6406:T2[])  [unwired: 11 in, 1 out]
                n3853 = case shown="1" w6405 {
                  tunnel: w6407 -> [w6416 w6417 _]
                  tunnel: [w6416 w6417 w6418] -> w6400
                  tunnel: w6406 -> [_ _ w6418]
                  frame 0, Default {
                  }
                  frame 1 {
                  }
                  frame 2 {
                  }
                }
                n3854 = for {
                  N: 12 -> [_]
                  tunnel: w6400 -> [w6425]
                  i -> [w6420]
                  # "①"
                  # "※複製コピーはこのケースで行う"
                  # "32回分"
                  # "比較する固定GNO"
                  n3855 = local read "メイン設定_設定 12"() -> (w6419:T2)
                  n3856 = Index Array(array=w6425, index=w6420) -> (element=w6424:T2)
                  n3857 = Unbundle By Name(w6419) -> ("ポートNo."=w6423:dbl)
                  n3858 = Unbundle By Name(w6424) -> ("ポートNo."=w6422:dbl)
                  n3859 = Equal?(x=w6423, y=w6422) -> (x = y?=w6421:bool)
                  n3860 = case shown="TRUE" w6421 {
                    tunnel: w6424 -> [_ w6427]
                    tunnel: w6420 -> [_ w6426]
                    frame False {
                    }
                    frame True {
                      n3861 = case shown="0, デフォルト" w6426 {
                        tunnel: w6427 -> [w6443 w6461 w6479 w6497 w6515 w6533 w6551 w6569 w6587 w6605 w6623 w6641]
                        tunnel: w6426 -> [w6442 w6460 w6478 w6496 w6514 w6532 w6550 w6568 w6586 w6604 w6622 w6640]
                        frame 0, Default {
                          w6433 = 2
                          # "B"
                          # "A"
                          # "csv作成の為表へクラスタ(実測値)書き込み"
                          # "⑤"
                          # "③"
                          # "④"
                          n3862 = local read "メインON/OFF_\n設定 1"() -> (w6444:T1)
                          n3863 = Unbundle By Name(w6444) -> ("使用ON/OFF"=w6440:bool)
                          n3864 = control-ref of="前回値転記用配列"() -> (w6438:refnum<vi>)
                          n3865 = local read "メイン設定_設定 1"() -> (w6445:T2)
                          n3866 = call "メイン_測定値配列_CSV転記サブ.vi"("メイン設定_設定入力"=w6445, "ループ反復数値入力"=w6442, "実測設定項目"=w6443, "使用ON/OFF"=w6440, "前回値転記用配列"=w6438) -> ("ループ反復数値出力"=w6441:i32, "メイン設定_設定出力"=w6439:T2)  [unwired: 5 in]
                          n3867 = local write "メイン設定_設定 1"(w6439) -> ()
                          n3868 = Add(x=2, y=w6441) -> (x+y=w6434:i32)
                          n3869 = Add(x=w6441, y=3) -> (x+y=w6432:i32)
                          n3870 = local read "csv作成表"() -> (w6428:string[][])
                          n3871 = Unbundle By Name(w6439) -> ("実測値(MAX)"=w6435:string, "実測値(MIN)"=w6436:string)
                          n3872 = Replace Array Subset(array=w6428, new element #1=w6435, index (row) #1=w6433, index (col) #1=w6434, new element #2=w6436, index (row) #2=w6433, index (col) #2=w6432) -> (w6430:string[][])
                          n3873 = Select(t=w6430, s=w6440, f=w6428) -> (s? t:f=w6431:string[][])
                          n3874 = local write "csv作成表"(w6431) -> ()
                        }
                        frame 1 {
                          w6451 = 2
                          # "B"
                          # "A"
                          # "csv作成の為表へクラスタ(実測値)書き込み"
                          # "⑤"
                          # "③"
                          # "④"
                          n3875 = local read "メインON/OFF_\n設定 2"() -> (w6462:T1)
                          n3876 = Unbundle By Name(w6462) -> ("使用ON/OFF"=w6458:bool)
                          n3877 = control-ref of="前回値転記用配列"() -> (w6456:refnum<vi>)
                          n3878 = local read "メイン設定_設定 2"() -> (w6463:T2)
                          n3879 = call "メイン_測定値配列_CSV転記サブ.vi"("メイン設定_設定入力"=w6463, "ループ反復数値入力"=w6460, "実測設定項目"=w6461, "使用ON/OFF"=w6458, "前回値転記用配列"=w6456) -> ("ループ反復数値出力"=w6459:i32, "メイン設定_設定出力"=w6457:T2)  [unwired: 5 in]
                          n3880 = local write "メイン設定_設定 2"(w6457) -> ()
                          n3881 = Add(x=3, y=w6459) -> (x+y=w6452:i32)
                          n3882 = Add(x=w6459, y=4) -> (x+y=w6450:i32)
                          n3883 = local read "csv作成表"() -> (w6446:string[][])
                          n3884 = Unbundle By Name(w6457) -> ("実測値(MAX)"=w6453:string, "実測値(MIN)"=w6454:string)
                          n3885 = Replace Array Subset(array=w6446, new element #1=w6453, index (row) #1=w6451, index (col) #1=w6452, new element #2=w6454, index (row) #2=w6451, index (col) #2=w6450) -> (w6448:string[][])
                          n3886 = Select(t=w6448, s=w6458, f=w6446) -> (s? t:f=w6449:string[][])
                          n3887 = local write "csv作成表"(w6449) -> ()
                        }
                        frame 2 {
                          w6469 = 2
                          # "B"
                          # "A"
                          # "csv作成の為表へクラスタ(実測値)書き込み"
                          # "⑤"
                          # "③"
                          # "④"
                          n3888 = local read "メインON/OFF_\n設定 3"() -> (w6480:T1)
                          n3889 = Unbundle By Name(w6480) -> ("使用ON/OFF"=w6476:bool)
                          n3890 = control-ref of="前回値転記用配列"() -> (w6474:refnum<vi>)
                          n3891 = local read "メイン設定_設定 3"() -> (w6481:T2)
                          n3892 = call "メイン_測定値配列_CSV転記サブ.vi"("メイン設定_設定入力"=w6481, "ループ反復数値入力"=w6478, "実測設定項目"=w6479, "使用ON/OFF"=w6476, "前回値転記用配列"=w6474) -> ("ループ反復数値出力"=w6477:i32, "メイン設定_設定出力"=w6475:T2)  [unwired: 5 in]
                          n3893 = local write "メイン設定_設定 3"(w6475) -> ()
                          n3894 = Add(x=4, y=w6477) -> (x+y=w6470:i32)
                          n3895 = Add(x=w6477, y=5) -> (x+y=w6468:i32)
                          n3896 = local read "csv作成表"() -> (w6464:string[][])
                          n3897 = Unbundle By Name(w6475) -> ("実測値(MAX)"=w6471:string, "実測値(MIN)"=w6472:string)
                          n3898 = Replace Array Subset(array=w6464, new element #1=w6471, index (row) #1=w6469, index (col) #1=w6470, new element #2=w6472, index (row) #2=w6469, index (col) #2=w6468) -> (w6466:string[][])
                          n3899 = Select(t=w6466, s=w6476, f=w6464) -> (s? t:f=w6467:string[][])
                          n3900 = local write "csv作成表"(w6467) -> ()
                        }
                        frame 3 {
                          w6487 = 2
                          # "B"
                          # "A"
                          # "csv作成の為表へクラスタ(実測値)書き込み"
                          # "⑤"
                          # "③"
                          # "④"
                          n3901 = local read "メインON/OFF_\n設定 4"() -> (w6498:T1)
                          n3902 = Unbundle By Name(w6498) -> ("使用ON/OFF"=w6494:bool)
                          n3903 = control-ref of="前回値転記用配列"() -> (w6492:refnum<vi>)
                          n3904 = local read "メイン設定_設定 4"() -> (w6499:T2)
                          n3905 = call "メイン_測定値配列_CSV転記サブ.vi"("メイン設定_設定入力"=w6499, "ループ反復数値入力"=w6496, "実測設定項目"=w6497, "使用ON/OFF"=w6494, "前回値転記用配列"=w6492) -> ("ループ反復数値出力"=w6495:i32, "メイン設定_設定出力"=w6493:T2)  [unwired: 5 in]
                          n3906 = local write "メイン設定_設定 4"(w6493) -> ()
                          n3907 = Add(x=5, y=w6495) -> (x+y=w6488:i32)
                          n3908 = Add(x=w6495, y=6) -> (x+y=w6486:i32)
                          n3909 = local read "csv作成表"() -> (w6482:string[][])
                          n3910 = Unbundle By Name(w6493) -> ("実測値(MAX)"=w6489:string, "実測値(MIN)"=w6490:string)
                          n3911 = Replace Array Subset(array=w6482, new element #1=w6489, index (row) #1=w6487, index (col) #1=w6488, new element #2=w6490, index (row) #2=w6487, index (col) #2=w6486) -> (w6484:string[][])
                          n3912 = Select(t=w6484, s=w6494, f=w6482) -> (s? t:f=w6485:string[][])
                          n3913 = local write "csv作成表"(w6485) -> ()
                        }
                        frame 4 {
                          w6505 = 2
                          # "B"
                          # "A"
                          # "csv作成の為表へクラスタ(実測値)書き込み"
                          # "⑤"
                          # "③"
                          # "④"
                          n3914 = local read "メインON/OFF_\n設定 5"() -> (w6516:T1)
                          n3915 = Unbundle By Name(w6516) -> ("使用ON/OFF"=w6512:bool)
                          n3916 = control-ref of="前回値転記用配列"() -> (w6510:refnum<vi>)
                          n3917 = local read "メイン設定_設定 5"() -> (w6517:T2)
                          n3918 = call "メイン_測定値配列_CSV転記サブ.vi"("メイン設定_設定入力"=w6517, "ループ反復数値入力"=w6514, "実測設定項目"=w6515, "使用ON/OFF"=w6512, "前回値転記用配列"=w6510) -> ("ループ反復数値出力"=w6513:i32, "メイン設定_設定出力"=w6511:T2)  [unwired: 5 in]
                          n3919 = local write "メイン設定_設定 5"(w6511) -> ()
